vi "Temporary Image Space.vi"(10 "Border Size":i32=3, 11 "Image Name":string) -> (3 "Image Out":T1)   [LabVIEW 2013]
doc: "VI is a clone so it can be called by different subvis and have unique image spaces for each. Creates an image space with the Image Name Passed in and the current VI name."
uses:
  <vilib>/vision/Image Controls.llb/IMAQ Image.ctl
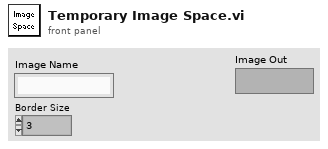
[diagram p1: front panel]
types:
  T1 = typedef "IMAQ Image.ctl" = refnum<image>
  T2 = typedef "Image Type" = u32
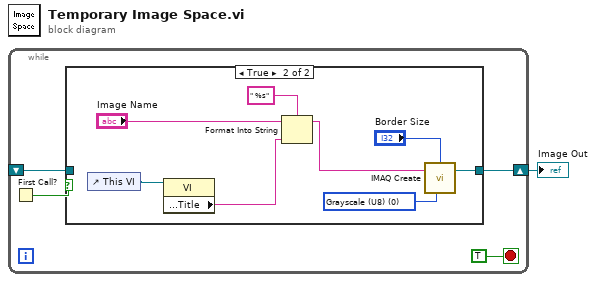
[diagram p0: block diagram]
diagram:
  n1 = while {
    shift-right: [w5] -> w1
    shift-left: _ -> [w2]
    stop <- TRUE stop-if-true
    n2 = First Call?() -> (First Call?: T/F=w3:bool)
    n3 = case shown="True" w3 {
      tunnel: [w6 w13] -> w5
      tunnel: w2 -> [w6 _]
      frame False {
      }
      frame True {
        w14 = T2 0 items=["Grayscale (U8)", "Grayscale (I16)", "Grayscale (SGL)", "Complex (CSG)", "RGB (U32)", "HSL (U32)", "RGB (U64)", "Grayscale (U16)"] ("Image Type")
        n4 = control-ref of="This VI"() -> (w12:refnum<vi>)
        n5 = property class="VI"(reference=w12) -> ("Front Panel.Title"=w9:string)  [unwired: 1 in, 2 out]
        n6 = Format Into String(format string=" %s", initial string="Image Name", w9) -> (resulting string=w8:string)  [unwired: 1 in, 1 out]
        n7 = call "IMAQ Create"("Border Size"="Border Size", "Image Name"=w8, "Image Type"=w14) -> ("New Image"=w13:T1)  [unwired: 2 in, 1 out]
      }
    }
  }
  "Image Out" <- w1
